vi "fileDatOpen.vi"(4 "transpose":bool, 5 "#frames":i32, 6 "frame0":i32, 7 "file path (use dialog)":path) -> (0 "folder":string, 1 "path":string, 2 "size(s)":dbl format="%.2f", 3 "output array":u16[][][](array[numeric]))   [LabVIEW 2017]
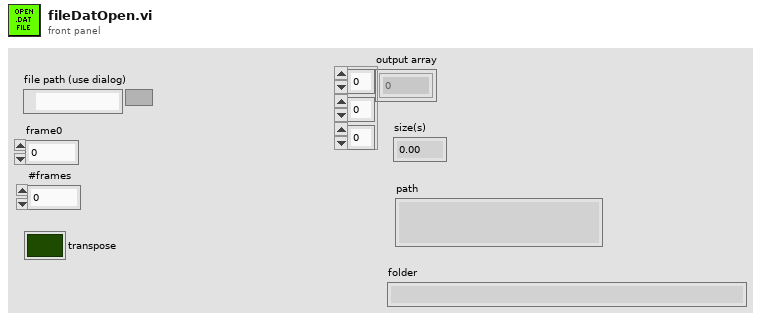
[diagram p1: front panel]
types:
  T1 = enum16{"big-endian, network order", "native, host order", "little-endian"}
  T2 = enum16{"open", "replace", "create", "open or create", "replace or create", "replace or create with confirmation"}
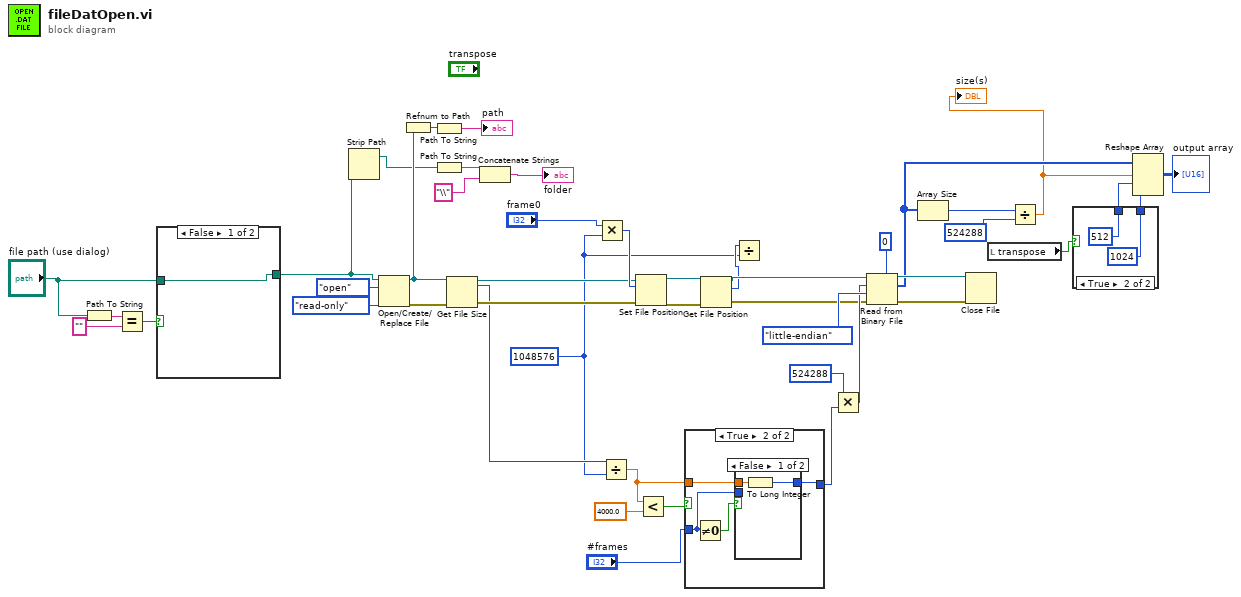
[diagram p0: block diagram]
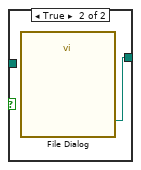
[diagram p2: hidden frame]
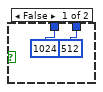
[diagram p3: hidden frame]
diagram:
  w20 = 1048576 ("x")
  n1 = Path To String(path="file path (use dialog)") -> (string=w11:string)
  n2 = Equal?(x=w11, y="") -> (x = y?=w9:bool)
  n3 = case shown="False" w9 {
    tunnel: [w46 w47] -> w7
    tunnel: "file path (use dialog)" -> [w46 _]
    frame False {
    }
    frame True {
      n4 = call "File Dialog"() -> ("selected path"=w47:path)  [unwired: 12 in, 3 out]
    }
  }
  n5 = Strip Path(path=w7) -> (stripped path=w6:path)  [unwired: 1 out]
  n6 = Open/Create/Replace File(file path (use dialog)=w7, operation (0:open)=T2."open", access (0:read/write)=enum16{"read/write", "read-only", "write-only"}."read-only") -> (refnum out=w15:refnum<file>, error out=w31:errorcluster)  [unwired: 3 in, 1 out]
  n7 = Refnum to Path(1:w15) -> (0:w16:path)
  n8 = Path To String(path=w16) -> (string=→"path":string)
  n9 = Path To String(path=w6) -> (string=w5:string)
  n10 = Get File Size(file=w15, error in=w31) -> (refnum out=w30:refnum<file>, size (in bytes)=w28:i64, 0:w29:errorcluster)
  n11 = Concatenate Strings(w5, "\\") -> (→"folder":string)
  n12 = Multiply(x="frame0", y=w20) -> (x*y=w32:i32)
  n13 = Divide(x=w28, y=w20) -> (x/y=w17:dbl)
  n14 = Set File Position(offset (in bytes) (0)=w32, refnum=w30, error in=w29) -> (refnum out=w25:refnum<file>, error out=w24:errorcluster)  [unwired: 1 in]
  n15 = Less?(x=w17, y=4000.0) -> (x < y?=w18:bool)
  n16 = case shown="True" w18 {
    tunnel: [w48 w51] -> w1
    tunnel: w17 -> [_ w52]
    tunnel: "#frames" -> [w48 w50]
    frame False {
    }
    frame True {
      n17 = Not Equal To 0?(x=w50) -> (x != 0?=w49:bool)
      n18 = case shown="False" w49 {
        tunnel: w52 -> [w54 _]
        tunnel: [w53 w55] -> w51
        tunnel: w50 -> [_ w55]
        frame False {
          n19 = To Long Integer(number=w54) -> (32bit integer=w53:i32)
        }
        frame True {
        }
      }
    }
  }
  n20 = Get File Position(4:w24, 7:w25) -> (0:w22:errorcluster, 2:w21:i64, 3:w23:refnum<file>)
  n21 = Divide(x=w21, y=w20) -> ()  [unwired: 1 out]
  n22 = Multiply(x=524288 ("y"), y=w1) -> (x*y=w34:i32)
  n23 = Read from Binary File(5:u16 0, 8:w22, 9:T1."little-endian" ("byte order (0:big-endian, network order)"), 10:w34, 11:w23) -> (0:w40:errorcluster, 2:w39:u16[], 3:w41:refnum<file>)  [unwired: 1 in, 1 out]
  n24 = Array Size(array=w39) -> (size(s)=w38:i32)
  n25 = Close File(refnum=w41, error in=w40) -> ()  [unwired: 2 out]
  n26 = local read "transpose"() -> (w13:bool)
  n27 = Divide(x=w38, y=524288) -> (x/y=w27:dbl)
  "size(s)" <- w27
  n28 = case shown="True" w13 {
    tunnel: [1024 ("dimension size") 512 ("dimension size")] -> w36
    tunnel: [512 ("dimension size") 1024 ("dimension size")] -> w35
    frame False {
    }
    frame True {
    }
  }
  n29 = Reshape Array(w39, w27, w36, w35) -> (→"output array":u16[][][])
